vi "Read Alarm Notifications.vi"(7 "Unit Address (1)":u8=1, 8 "error in (no error)":errorcluster, 11 "VISA resource name":refnum<visa-resource-name>) -> (0 "error out":errorcluster, 1 "Any Alarm":bool, 2 "New Alarm":bool, 3 "VISA resource name out":refnum<visa-resource-name>)   [LabVIEW 2014, in "Eurotherm 35xx Series.lvlib"]
doc: "This VI reads Alarm notification values."
uses:
  <instrlib>/Eurotherm 35xx Series/Eurotherm 35xx Series.lvlib
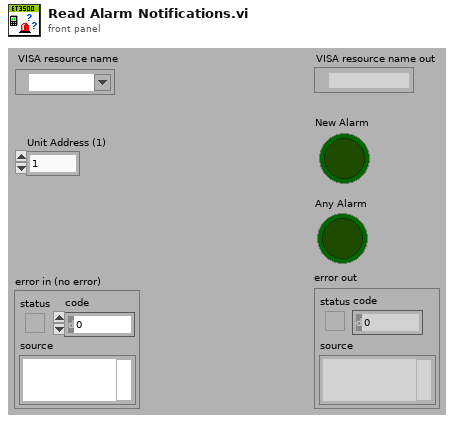
[diagram p1: front panel]
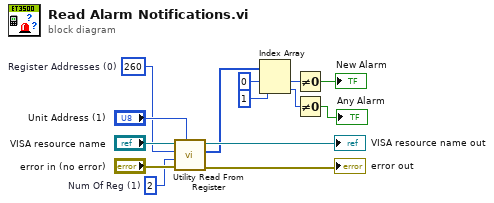
[diagram p0: block diagram]
diagram:
  w9 = u16 2  # Num Of Reg (1)
  w4 = 260  # Register Addresses (0)
  n1 = call <instrlib>:"Utility Read From Register.vi"("Unit Address (1)"="Unit Address (1)", "error in (no error)"="error in (no error)", "Num Of Reg (1)"=w9, "Register Address (0)"=w4, "VISA resource name"="VISA resource name") -> ("error out"=→"error out":errorcluster, "Data"=w8:i16[], "VISA resource name out"=→"VISA resource name out":refnum<visa-resource-name>)  [unwired: 4 in]
  n2 = Index Array(array=w8, index #1=0 ("index"), index #2=1 ("index")) -> (element #1=w6:i16, element #2=w2:i16)
  n3 = Not Equal To 0?(x=w6) -> (x != 0?=→"New Alarm":bool)
  n4 = Not Equal To 0?(x=w2) -> (x != 0?=→"Any Alarm":bool)
